vi "Launch Actor.vi"(6 "Open Actor Core front panel? (F)":bool, 8 "error in (no error)":errorcluster, 10 "Actor-to-Caller Enqueuer":refnum<class "Message Enqueuer.lvclass">, 11 "Actor":refnum<class "Actor.lvclass">) -> (0 "error out":errorcluster, 3 "Caller-To-Actor Enqueuer":refnum<class "Message Enqueuer.lvclass">)   [LabVIEW 2013, in "Actor Framework.lvlib" / "Actor.lvclass"]
doc: "(<B>Filename</B>: Actor Framework.lvlib:Actor.lvclass:Launch Actor.vi)\n\nLaunches a top-level VI that handles messages for an actor and starts this actor's tasks. This VI returns a reference to the queue you use to send messages to the actor.\n\nThis VI requires the <B>Actor-to-Caller Enqueuer</B> input, which is the reference that allows the launched actor to communicate with the caller. If you are launching the top-level actor, use the Read Enqueuer method to obtain this reference. If you are launching a nested actor, use the Read Self Enqueuer method instead."
uses:
  <vilib>/ActorFramework/Actor/Actor.lvclass
  <vilib>/ActorFramework/Message Enqueuer/Message Enqueuer.lvclass
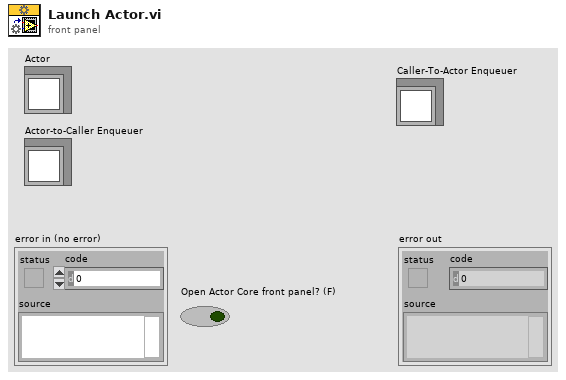
[diagram p1: front panel]
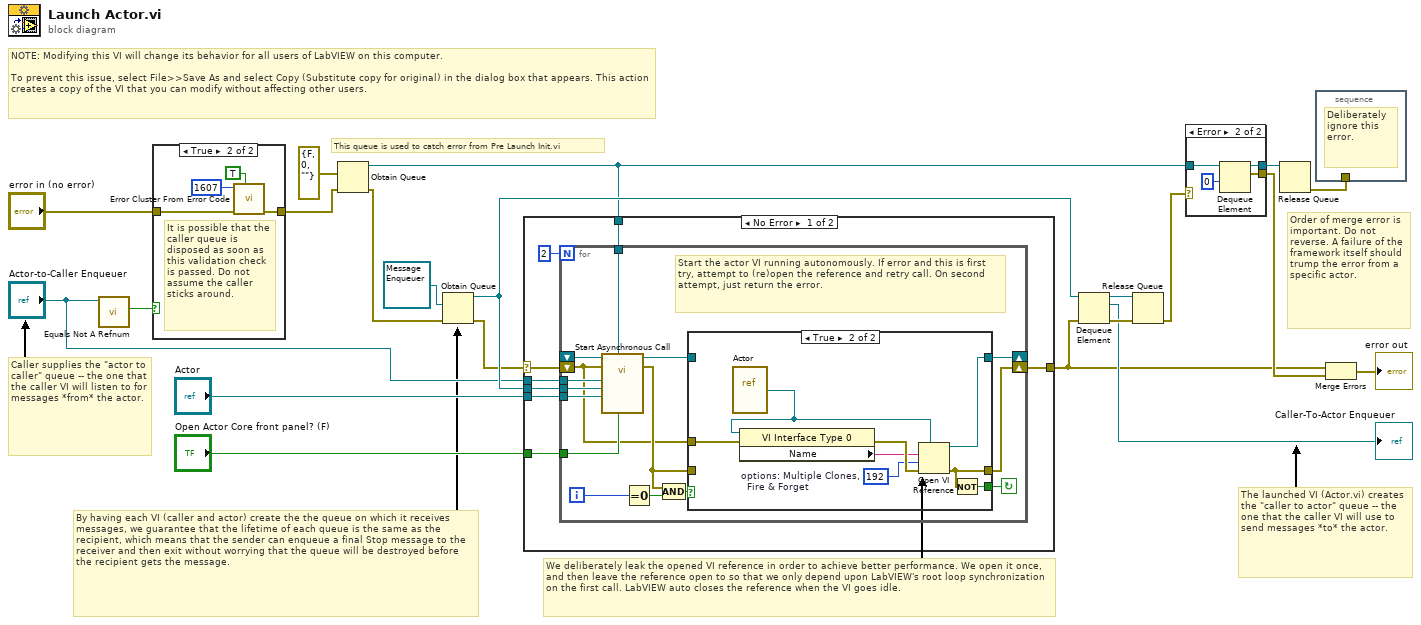
[diagram p0: block diagram]
diagram:
  # "Caller supplies the \"actor to caller\" queue -- the one that the caller VI will listen to for messages *from* the actor."
  # "We deliberately leak the opened VI reference in order to achieve better performance. We open it once, and then leave the reference open to so that we only depend upon LabVIEW's root loop synchronization on the first call. LabVIEW auto closes the reference when the VI goes idle."
  # "By having each VI (caller and actor) create the the queue on which it receives messages, we guarantee that the lifetime of each queue is the same as the recipient, which means that the sender can enqueue a final Stop message to the receiver and then exit without worrying that the queue will be destroyed before the recipient gets the message."
  # "This queue is used to catch error from Pre Launch Init.vi"
  # "Order of merge error is important. Do not reverse. A failure of the framework itself should trump the error from a specific actor."
  # "NOTE: Modifying this VI will change its behavior for all users of LabVIEW on this computer.\n\nTo prevent this issue, select File>>Save As and select Copy (Substitute copy for original) in the dialog box that appears. This action creates a copy of the VI that you can modify without affecting other users."
  # "The launched VI (Actor.vi) creates the \"caller to actor\" queue -- the one that the caller VI will use to send messages *to* the actor."
  n1 = call <vilib>:"Equals Not A Refnum.vi"("Message Enqueuer"="Actor-to-Caller Enqueuer") -> ("Not a refnum?"=w16:bool)  [unwired: 10 in]
  n2 = case shown="True" w16 {
    tunnel: "error in (no error)" -> [w22 w26]
    tunnel: [w22 w25] -> w3
    frame False {
    }
    frame True {
      # "It is possible that the caller queue is disposed as soon as this validation check is passed. Do not assume the caller sticks around."
      n3 = call <vilib>:"Error Cluster From Error Code.vi"("show call chain? (False)"=TRUE, "error in (no error)"=w26, "error code (0)"=1607) -> ("error out"=w25:errorcluster)  [unwired: 6 in]
    }
  }
  n4 = Obtain Queue(element data type=errorcluster {"status"=FALSE, "code"=0, "source"=""} ("Error"), error in (no error)=w3) -> (queue out=w9:refnum<queue>, error out=w11:errorcluster)  [unwired: 3 in, 1 out]
  n5 = Obtain Queue(element data type=refnum<class "Message Enqueuer.lvclass"> refnum ("Message Enqueuer"), error in (no error)=w11) -> (queue out=w14:refnum<queue>, error out=w5:errorcluster)  [unwired: 3 in, 1 out]
  n6 = case shown="No Error" w5 {
    selector: w5 -> [w27 w60]
    tunnel: "Actor" -> [w34 _]
    tunnel: "Actor-to-Caller Enqueuer" -> [w33 _]
    tunnel: "Open Actor Core front panel? (F)" -> [w32 _]
    tunnel: w14 -> [w31 _]
    tunnel: w9 -> [w30 _]
    tunnel: [w28 w60] -> w4
    frame No Error {
      n7 = for {
        N: 2 -> [_]
        tunnel: w34 -> [w49]
        tunnel: w33 -> [w48]
        tunnel: w32 -> [w47]
        tunnel: w31 -> [w46]
        tunnel: w30 -> [w45]
        shift-right: [w44] -> _
        shift-left: _ -> [w43]
        shift-right: [w41] -> w28
        shift-left: w27 -> [w35]
        i -> [w38]
        stop <- w36 continue-if-true
        # "Start the actor VI running autonomously. If error and this is first try, attempt to (re)open the reference and retry call. On second attempt, just return the error."
        n8 = call-by-ref "Start Asynchronous Call"(reference=w43, error in=w35, "Open Actor Core front panel? (F)"=w47, "error feedback"=w45, "Actor"=w49, "queue of queues"=w46, "Send Queue"=w48) -> (reference out=w42:refnum<vi>, error out=w37:errorcluster)  [unwired: 7 in]
        n9 = Equal To 0?(x=w38) -> (x = 0?=w39:bool)
        n10 = Compound Arithmetic op=AND(w37, w39) -> (w40:bool)
        n11 = case shown="True" w40 {
          tunnel: [w51 w56] -> w44
          tunnel: [w50 w53] -> w41
          tunnel: w42 -> [w51 _]
          tunnel: w37 -> [w50 _]
          tunnel: [_ w54] -> w36
          tunnel: w35 -> [_ w52]
          frame False {
          }
          frame True {
            w57 = 192  # options: Multiple Clones,   Fire & Forget
            n12 = vi-ref <vilib>:"Actor.vi"() -> (w55:refnum<vi>)
            n13 = property class="VI Interface Type 0"(reference=w55, error in=w52) -> (error out=w59:errorcluster, "Name"=w58:string)  [unwired: 1 out]
            n14 = Open VI Reference(type specifier VI Refnum (for type only)=w55, vi path=w58, options=w57, error in (no error)=w59) -> (vi reference=w56:refnum<vi>, error out=w53:errorcluster)  [unwired: 2 in]
            n15 = Not(x=w53) -> (.not. x?=w54:bool)
          }
        }
      }
    }
    frame Error {
    }
  }
  n16 = Dequeue Element(queue=w14, error in (no error)=w4) -> (queue out=w20:refnum<queue>, element=→"Caller-To-Actor Enqueuer":refnum<class "Message Enqueuer.lvclass">, error out=w19:errorcluster)  [unwired: 1 in, 1 out]
  n17 = Release Queue(queue=w20, error in (no error)=w19) -> (error out=w7:errorcluster)  [unwired: 1 in, 2 out]
  n18 = case shown="Error" w7 {
    selector: w7 -> [w62 _]
    tunnel: w9 -> [w61 w66]
    tunnel: [w62 w64] -> w8
    tunnel: [w61 w63] -> w6
    frame No Error {
    }
    frame Error {
      n19 = Dequeue Element(queue=w66, timeout in ms (-1)=0) -> (queue out=w63:refnum<queue>, element=w64:errorcluster)  [unwired: 1 in, 2 out]
    }
  }
  n20 = Release Queue(queue=w6) -> (error out=w1:errorcluster)  [unwired: 2 in, 2 out]
  n21 = stacked-sequence {
    tunnel: w1 -> [_]
    frame #0 {
      # "Deliberately ignore this error."
    }
  }
  n22 = Merge Errors(w4, w8) -> (→"error out":errorcluster)
